vi "EnqueVa(ErrorSupport).vi"(7 "コマンド":string, 8 "エラー入力（エラーなし）":errorcluster, 9 "タイムアウト（ms）（-1）":i32=-1, 10 "バリアント":variant, 11 "queVariant":refnum<queue>) -> (0 "エラー出力":errorcluster, 1 "timeout/overflow?":bool, 3 "queVariant(copy)":refnum<queue>)   [LabVIEW 2014]
uses:
  QueData.ctl
panel:
  in  "モード(Normal)":enum16{"Normal", "Lossy", "OppositeEnd"}(ring)
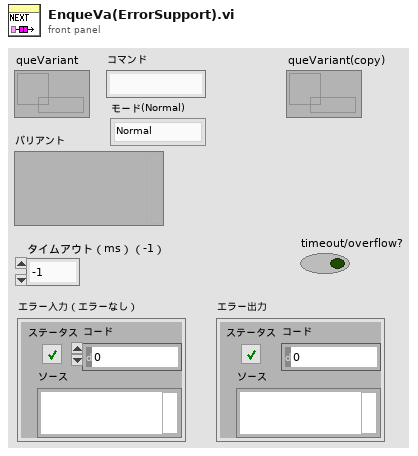
[diagram p1: front panel]
types:
  T1 = typedef "QueData.ctl" = cluster{"コマンド":string, "バリアント":variant}
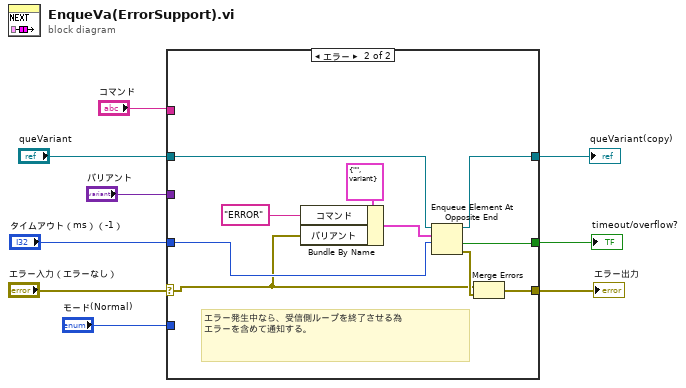
[diagram p0: block diagram]
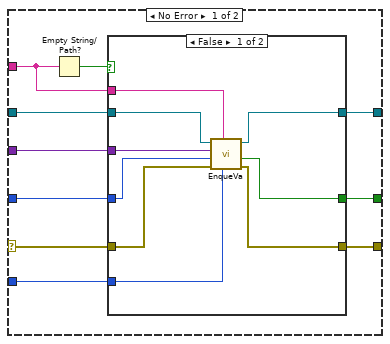
[diagram p2: hidden frame]
diagram:
  n1 = case shown="エラー" "エラー入力（エラーなし）" {
    selector: "エラー入力（エラーなし）" -> [w16 w31]
    tunnel: "queVariant" -> [w18 w33]
    tunnel: [w17 w34] -> w8
    tunnel: [w15 w37] -> w6
    tunnel: [w13 w36] -> w5
    tunnel: "タイムアウト（ms）（-1）" -> [w14 w35]
    tunnel: "コマンド" -> [w12 _]
    tunnel: "バリアント" -> [w11 _]
    tunnel: "モード(Normal)" -> [w10 _]
    frame No Error {
      n2 = Empty String/Path?(string/path=w12) -> (empty?=w19:bool)
      n3 = case shown="FALSE" w19 {
        tunnel: w18 -> [w27 w30]
        tunnel: [w25 w30] -> w17
        tunnel: w16 -> [w23 w29]
        tunnel: [w22 w29] -> w15
        tunnel: w11 -> [w28 _]
        tunnel: w14 -> [w24 _]
        tunnel: w12 -> [w26 _]
        tunnel: [w21 _] -> w13
        tunnel: w10 -> [w20 _]
        frame False {
          n4 = call "EnqueVa.vi"("モード(Normal)"=w20, "コマンド"=w26, "エラー入力（エラーなし）"=w23, "タイムアウト（ms）（-1）"=w24, "バリアント"=w28, "queVariant"=w27) -> ("エラー出力"=w22:errorcluster, "timeout/overflow?"=w21:bool, "queVariant(copy)"=w25:refnum<queue>)  [unwired: 3 in]
        }
        frame True {
        }
      }
    }
    frame Error {
      # "エラー発生中なら、受信側ループを終了させる為\nエラーを含めて通知する。"
      n5 = Bundle By Name(cluster=T1 {"コマンド"="", "バリアント"=variant} ("要素"), "コマンド"="ERROR", "バリアント"=w31) -> (w39:T1)
      n6 = Enqueue Element At Opposite End(queue=w33, element=w39, timeout in ms (-1)=w35) -> (queue out=w34:refnum<queue>, timed out?=w36:bool, error out=w38:errorcluster)  [unwired: 1 in]
      n7 = Merge Errors(w31, w38) -> (w37:errorcluster)
    }
  }
  "エラー出力" <- w6
  "queVariant(copy)" <- w8
  "timeout/overflow?" <- w5
